vi "pp_trialTypes_selectTrial.vi"(7 "Trial Code":i32, 8 "Error In":errorcluster, 11 "Trial Types":T2(array[cluster]) {"Stim P2" min=0.0; "Trial Weight" step=1; "Stim P1" min=0.0; "Stim Dur (s)" min=0.0; "Trial Code" min=1 step=1}) -> (0 "Error Out":errorcluster, 3 "Current/Cued Trial":T1={"Trial Code"=1, "Trial Type"=enum."GO", "Trial Weight"=0, "Stim Type"=enum."FM Sweep", "Stim Dur (s)"=2.0, "Stim P1"=4.0, "Stim P2"=0.0} {"Stim P2" min=0.0; "Trial Weight" step=1; "Stim P1" min=0.0; "Stim Dur (s)" min=0.0; "Trial Code" min=1 step=1})   [LabVIEW 2013]
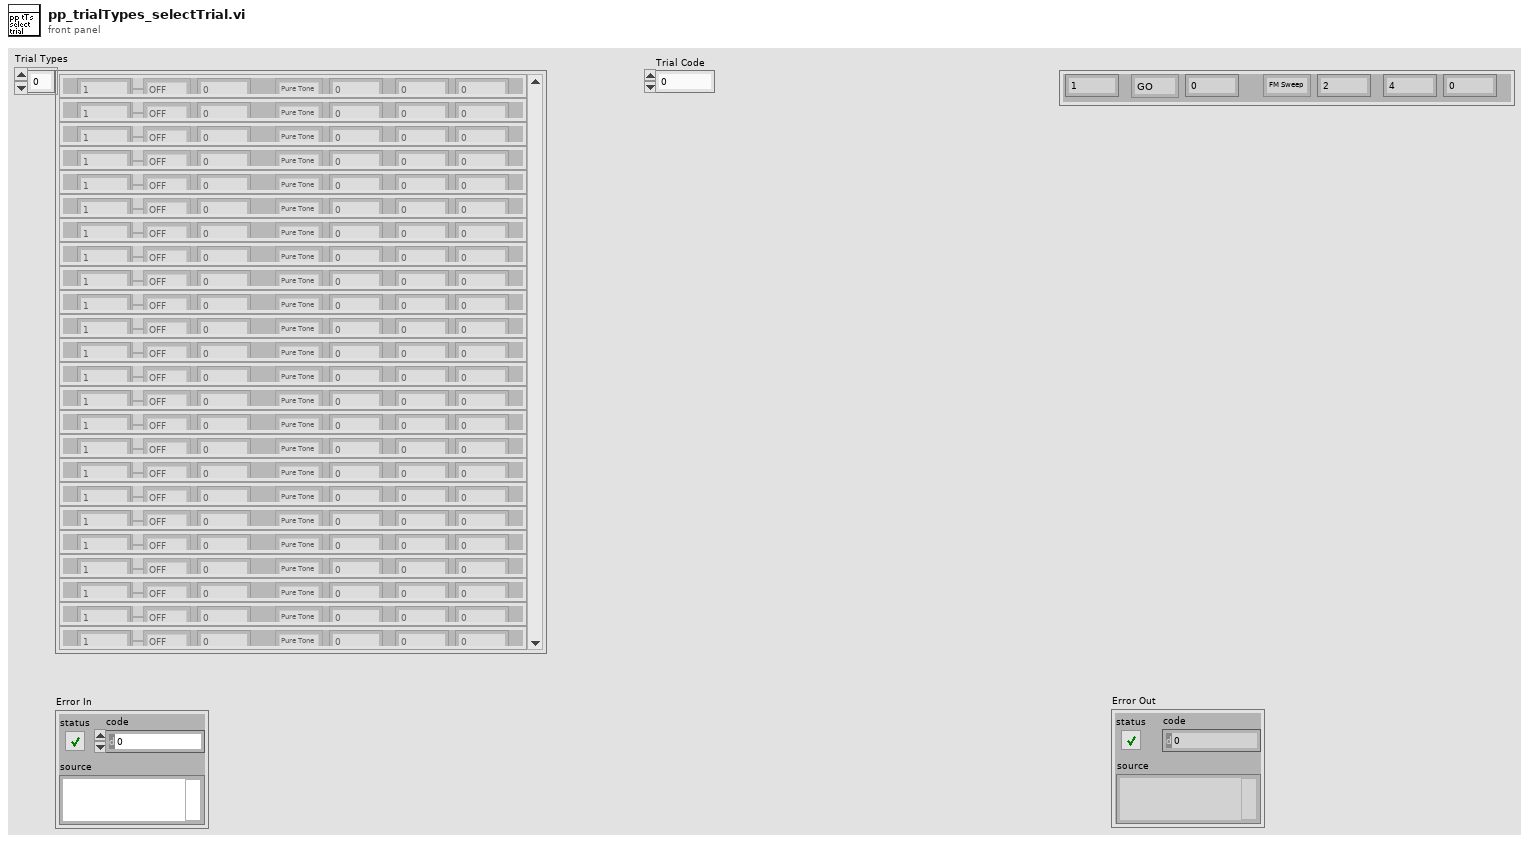
[diagram p1: front panel]
types:
  T1 = cluster{"Trial Code":u16, "Trial Type":enum16{"OFF", "GO", "NOGO", "TEST"}, "Trial Weight":u32, "Stim Type":enum16{"Pure Tone", "FM Sweep"}, "Stim Dur (s)":dbl, "Stim P1":dbl, "Stim P2":dbl}
  T2 = cluster{"Trial Code":u16, "Trial Type":enum16{"OFF", "GO", "NOGO", "TEST"}, "Trial Weight":u32, "Stim Type":enum16{"Pure Tone", "FM Sweep"}, "Stim Dur (s)":dbl, "Stim P1":dbl, "Stim P2":dbl}[]
  T3 = cluster{"Trial Code":bool, "Trial Type":bool, "Trial Weight":bool, "Stim Type":bool, "Stim Dur (s)":bool, "Stim P1":bool, "Stim P2":bool}
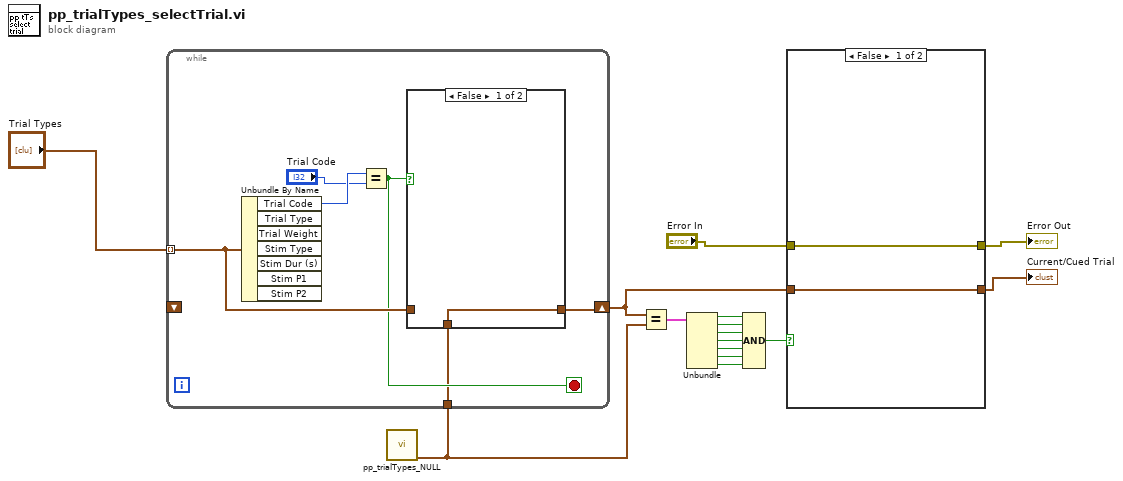
[diagram p0: block diagram]
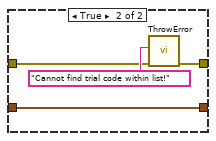
[diagram p2: hidden frame]
diagram:
  n1 = call "pp_trialTypes_NULL.vi"() -> ("Cluster"=w14:T1)  [unwired: 10 in, 1 out]
  n2 = while {
    tunnel: "Trial Types" -> [w19] mode=indexing
    shift-right: [w18] -> w4
    shift-left: _ -> [_]
    tunnel: w14 -> [w16]
    stop <- w17 stop-if-true
    n3 = Unbundle By Name(w19) -> ("Trial Code"=w21:u16)  [unwired: 6 out]
    n4 = Equal?(x=w21, y="Trial Code") -> (x = y?=w17:bool)
    n5 = case shown="False" w17 {
      tunnel: w19 -> [_ w23]
      tunnel: [w22 w23] -> w18
      tunnel: w16 -> [w22 _]
      frame False {
      }
      frame True {
      }
    }
  }
  n6 = Equal?(x=w4, y=w14) -> (x = y?=w13:T3)
  n7 = Unbundle(w13) -> ("Trial Code"=w12:bool, "Trial Type"=w11:bool, "Trial Weight"=w10:bool, "Stim Type"=w9:bool, "Stim Dur (s)"=w8:bool, "Stim P1"=w7:bool, "Stim P2"=w6:bool)
  n8 = Compound Arithmetic op=AND(w12, w11, w10, w9, w8, w7, w6) -> (w5:bool)
  n9 = case shown="False" w5 {
    tunnel: w4 -> [w24 w29]
    tunnel: [w24 w29] -> w3
    tunnel: "Error In" -> [w25 w27]
    tunnel: [w25 w26] -> w1
    frame False {
    }
    frame True {
      n10 = call "ThrowError.vi"("error in (no error)"=w27, "Error Message"="Cannot find trial code within list!") -> ("error out"=w26:errorcluster)  [unwired: 8 in, 1 out]
    }
  }
  "Current/Cued Trial" <- w3
  "Error Out" <- w1
